vi "Poll Position.vi"(8 "error in (no error)":errorcluster, 10 "Hardware State":T1) -> (0 "error out":errorcluster, 1 "XYZ Microns":dbl[](array[numeric]), 2 "Hardware State Out":T1)   [LabVIEW 2015, in "XYZStage.lvlib"]
uses:
  XYZStage.lvlib
  XYZStage State.ctl
  XYZStage Loop State.ctl
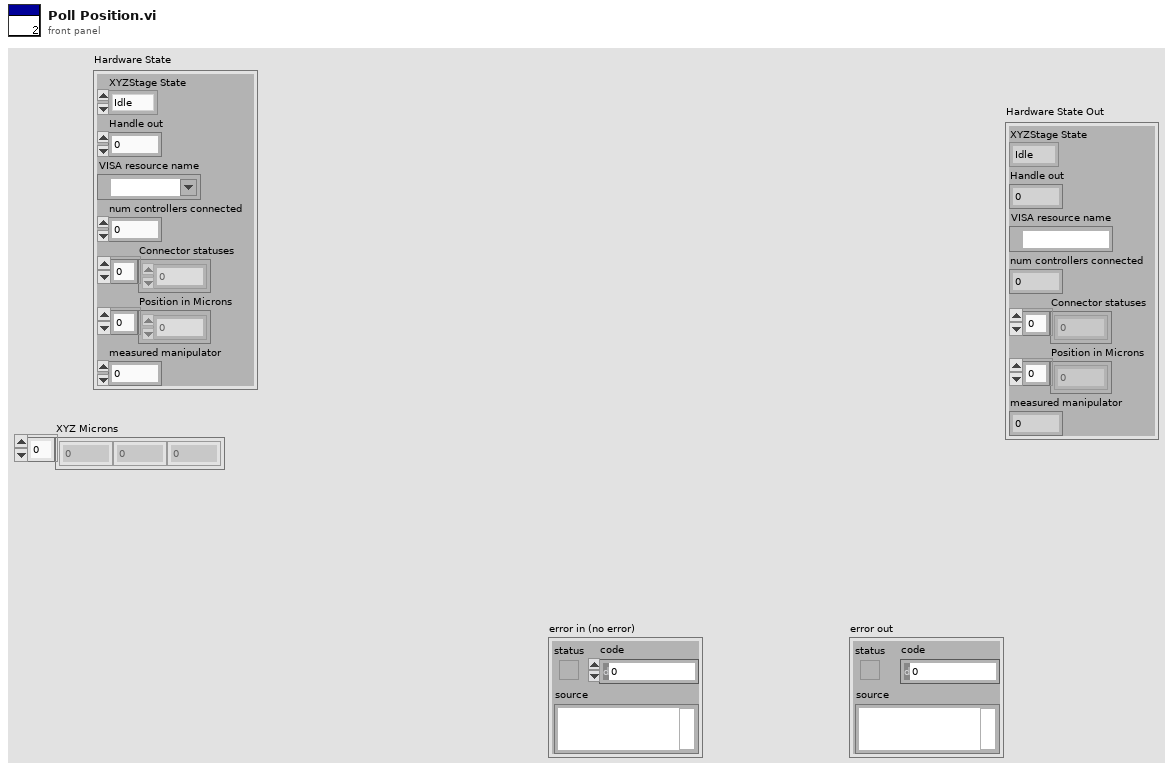
[diagram p1: front panel]
types:
  T1 = typedef "XYZStage.lvlib/XYZStage State.ctl" = cluster{"XYZStage State":T2, "Handle out":u32, "VISA resource name":refnum<visa-resource-name>, "num controllers connected":u8, "Connector statuses":u8[], "Position in Microns":dbl[], "measured manipulator":u8}
  T2 = typedef "XYZStage.lvlib/XYZStage Loop State.ctl" = enum16{"Idle", "Connected", "Moving"}
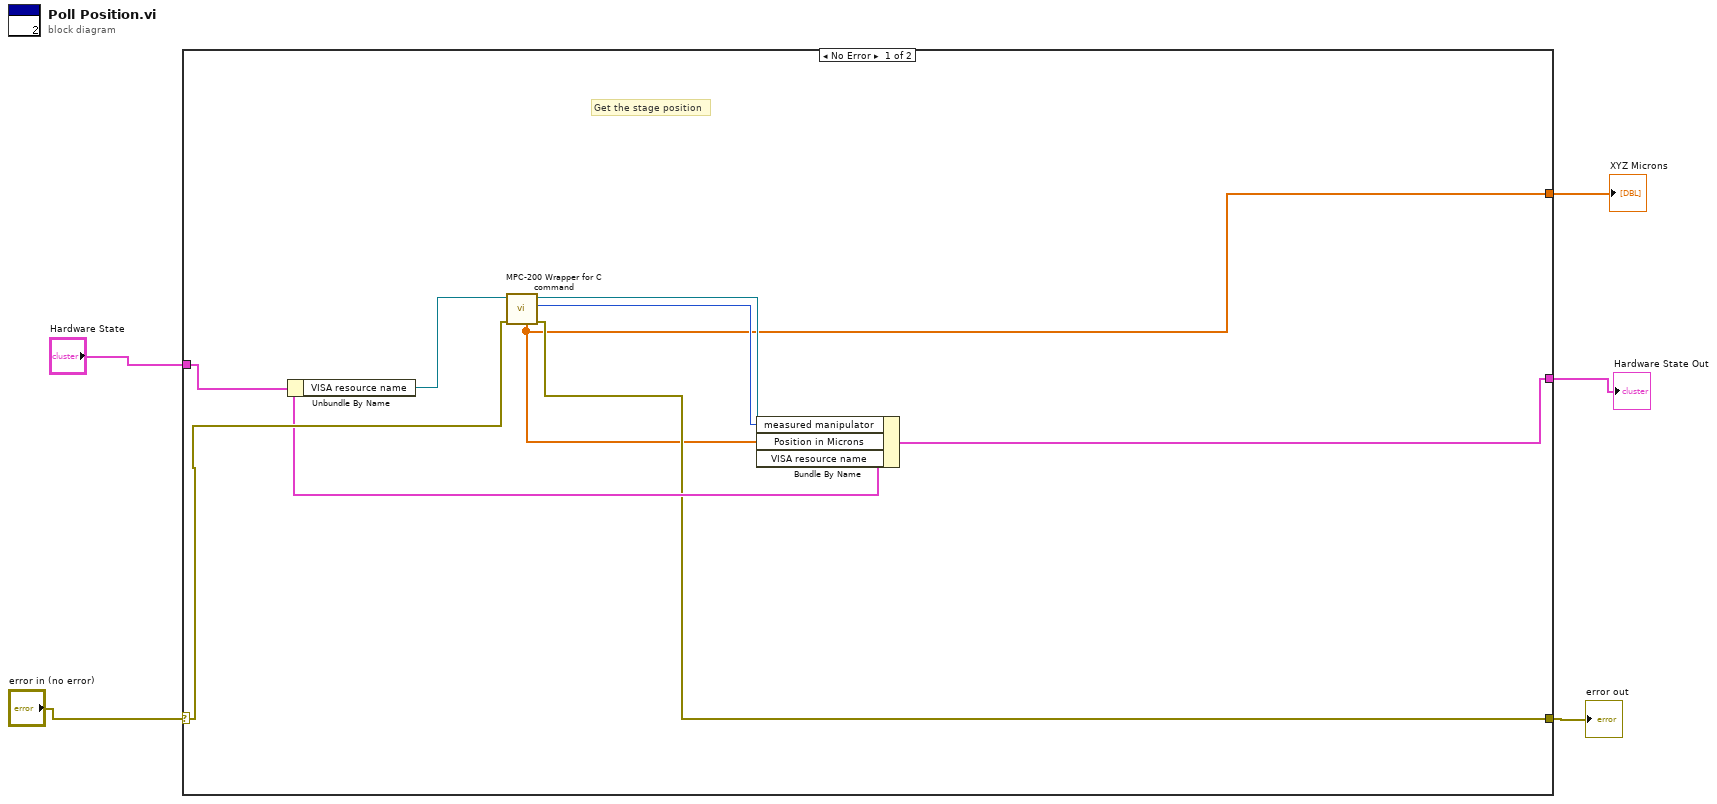
[diagram p0: block diagram]
diagram:
  n1 = case shown="No Error" "error in (no error)" {
    selector: "error in (no error)" -> [w10 w15]
    tunnel: [w7 w15] -> w4
    tunnel: [w8 w14] -> w3
    tunnel: "Hardware State" -> [w9 w14]
    tunnel: [w6 _] -> w1
    frame No Error {
      # "Get the stage position"
      n2 = Unbundle By Name(w9) -> ("VISA resource name"=w13:refnum<visa-resource-name>)
      n3 = call "MPC-200 Wrapper for C command.vi"("error in (no error)"=w10, "VISA resource name in"=w13) -> ("error out"=w7:errorcluster, "Manipulator Number"=w11:u8, "VISA resource name out"=w12:refnum<visa-resource-name>, "XYZ Microns"=w6:dbl[])  [unwired: 5 in, 1 out]
      n4 = Bundle By Name(cluster=w9, "measured manipulator"=w11, "Position in Microns"=w6, "VISA resource name"=w12) -> (w8:T1)
    }
    frame Error {
    }
  }
  "error out" <- w4
  "Hardware State Out" <- w3
  "XYZ Microns" <- w1
